vi "Firmware Wizard.vi"() -> ()   [LabVIEW 2020, in "LMH-LINX.lvlib"]
doc: "Wizard for uploading firmware to LINX devices."
uses:
  <vilib>/MakerHub/LINX/LMH-LINX.lvlib
  <vilib>/MakerHub/LINX/Private/Type Defs/Device Family.ctl
  <vilib>/MakerHub/LINX/Private/Type Defs/Devices/Device Type.ctl
  <vilib>/MakerHub/LINX/Private/Device/Type Defs/Wifi Config.ctl
  <vilib>/MakerHub/LINX/Private/Type Defs/WIFI Security Type.ctl
  <vilib>/MakerHub/LINX/Private/Type Defs/Deploy Firmware State.ctl
  <vilib>/MakerHub/LINX/Private/Type Defs/All Firmware Data FGV States.ctl
  <vilib>/MakerHub/LINX/Private/Device/Type Defs/TCP Config.ctl
  <vilib>/MakerHub/LINX/Private/Device/Type Defs/Firmware Interface.ctl
  <vilib>/MakerHub/Toolbox/LMH-Toolbox.lvlib
  <vilib>/MakerHub/LINX/Private/Device/Device.lvlib
panel:
  out "Error Out":errorcluster
  out "Log Path":path
  in  "Device Family Enum":T1 items=["National Instruments", "Digilent", "Arduino"]
  in  "Error In":errorcluster
  out "Tab Control":T2(tab)=enum."Device"
  in  "Firmware Available?":string
  in  "Settings Button":bool
  out "Device Image":picture
  in  "Device Help":bool
  in  "Device Type":T3=4 items=["Arduino Leonardo", "Arduino Mega2560", "Arduino Nano", "Arduino Pro Micro", "Arduino Uno"]
  in  "Device Family":T1 items=["Arduino", "Digilent", "PJRC", "Sparkfun"]
  in  "Device Cancel":bool
  in  "Device Next":bool
  in  "Firmware Upload Method":u16(ring) items=["Serial / USB"]
  in  "Config Message":string
  in  "Int Help":bool
  in  "Int Previous":bool
  in  "Int Cancel":bool
  in  "Int Next":bool
  out "Interface Config":enum32{"N/A", "Serial / USB", "USB", "TCP"}(tab)=enum."Serial / USB"
  in  "Upload COM Port":refnum<visa-resource-name>="ASRL1::INSTR"
  out "Firmware Configuration":enum32{"Serial", "Ethernet", "WIFI"}(tab)=enum."WIFI"
  in  "Port":u16=927
  in  "IP Address":string="192.168.1.27"
  in  "Wifi Configuration":T4
  in  "FWV Help":bool
  in  "FWV Cancel":bool
  in  "FWV Next":bool
  in  "FWV Previous":bool
  in  "Firmware Version":u16(ring) items=["LINX - Serial / USB"]
  in  "Upload Type":u16(ring) items=["Pre-Built Firmware", "Build with Arduino IDE"]
  in  "Firmware Description":string
  out "Deploy Progress Note":string
  in  "Deploy  Progress Bar":u8(slide) scale=0.0..100.0
  in  "View Log":bool
  in  "LINX Forum Link":string="www.labviewmakerhub.com/forums/linx"
  in  "LINX Landing Page Link":string="www.labviewmakerhub.com/linx"
  in  "Summary Launch Example":bool
  in  "Summary Text":string
  in  "Summary Next":bool
  in  "Summary Help":bool
  # "Ethernet Settings"
  # "WIFI Settings"
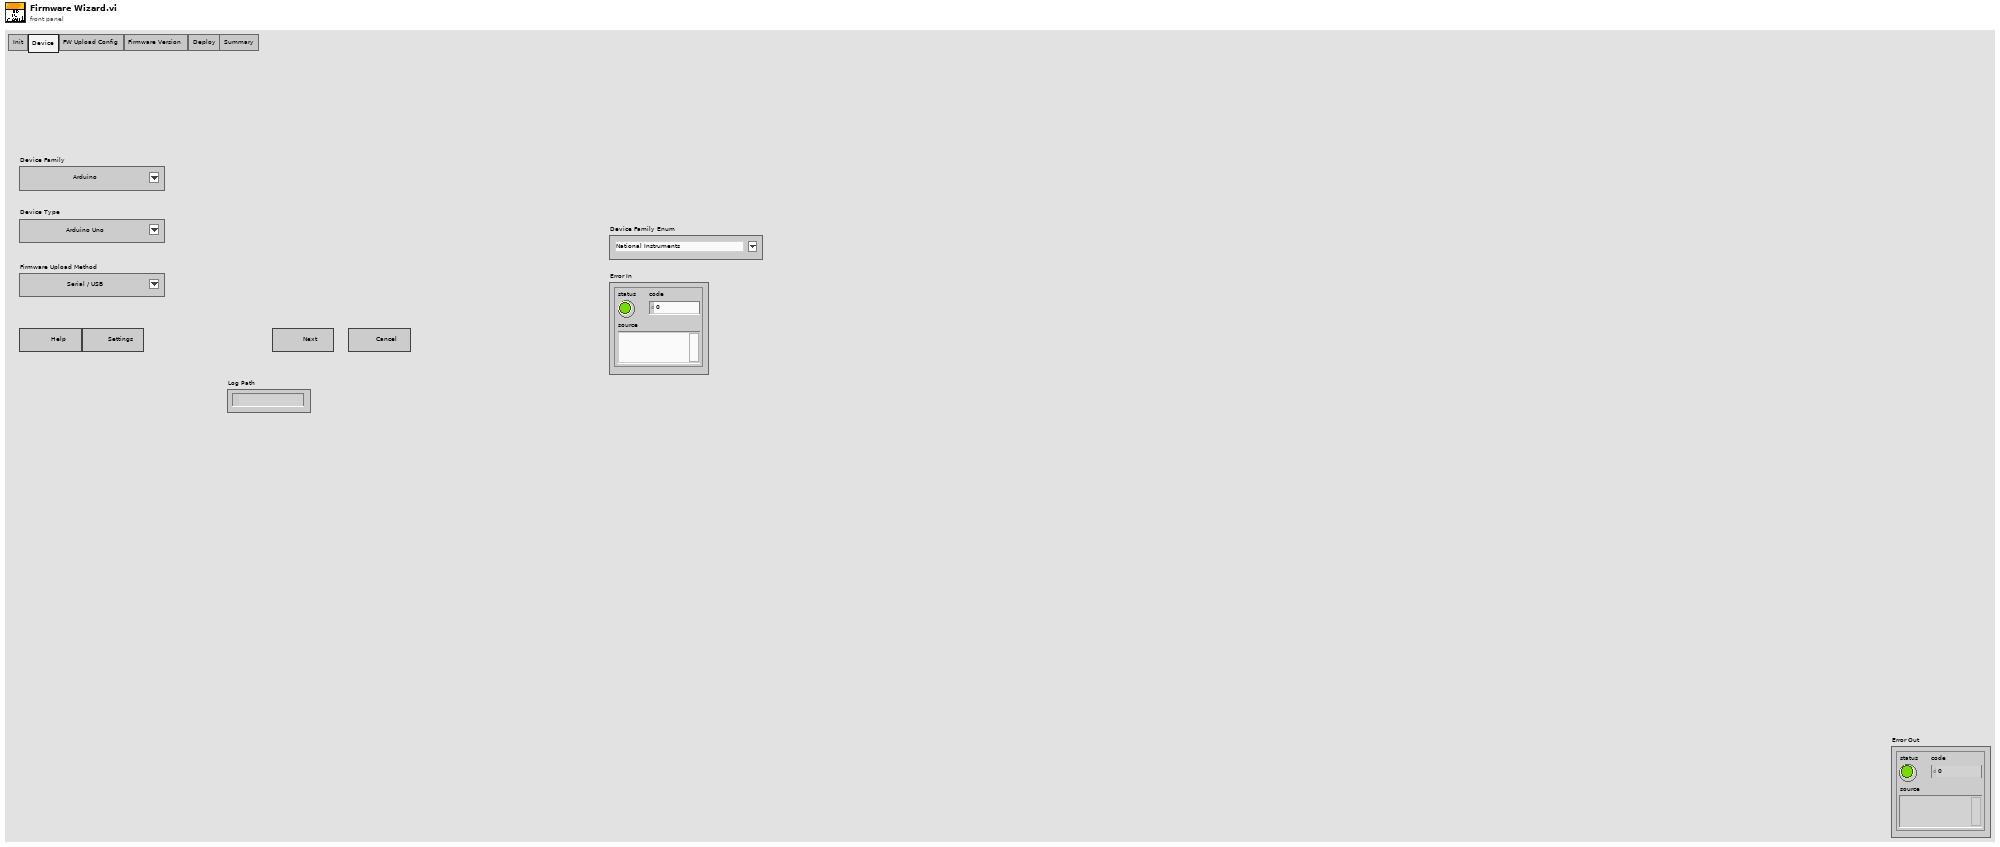
[diagram p1: front panel]
types:
  T1 = typedef "LMH-LINX.lvlib/Device Family.ctl" = u8
  T2 = enum32{"Init", "Device", "FW Upload Config", "Firmware Version", "Deploy", "Summary"}
  T3 = typedef "LMH-LINX.lvlib/Device Type.ctl" = u16
  T4 = typedef "LMH-LINX.lvlib/Device.lvlib/Wifi Config.ctl" = cluster{"SSID":string, "IP Address":string, "Port":u16, "WIFI Security Type":T5, "Password":string}
  T5 = typedef "LMH-LINX.lvlib/WIFI Security Type.ctl" = enum8{"None", "WPA2 Password", "WPA2 Key", "WEP40", "WEP104"}
  T6 = typedef "LMH-LINX.lvlib/Deploy Firmware State.ctl" = enum32{"Init", "Device", "FW Upload Config", "Firmware Version", "Deploy", "Summary"}
  T7 = typedef "LMH-LINX.lvlib/All Firmware Data FGV States.ctl" = enum16{"Set", "Get"}
  T8 = enum8{"Enabled", "Disabled", "Disabled and Grayed Out"}
  T9 = typedef "LMH-LINX.lvlib/Firmware Interface.ctl" = enum32{"Serial ", "Ethernet", "WIFI"}
  T10 = typedef "LMH-LINX.lvlib/Device.lvlib/TCP Config.ctl" = cluster{"IP Address":string, "Port":u16}
  T11 = typedef "LMH-LINX.lvlib/Device Firmware.ctl" = cluster{"Firmware Name":string, "Firmware Path":path, "Description":string, "LINX Interface":string, "Flash Util Working Dir":path, "Flash Util Name":string, "Flash Util Args":string, "Flash Timeout (ms)":i32, "Pre-Built Firmware":string, "Build with Arduino IDE":string}
  T12 = enum16{"Left Button", "Center Button", "Right Button", "Window Close"}
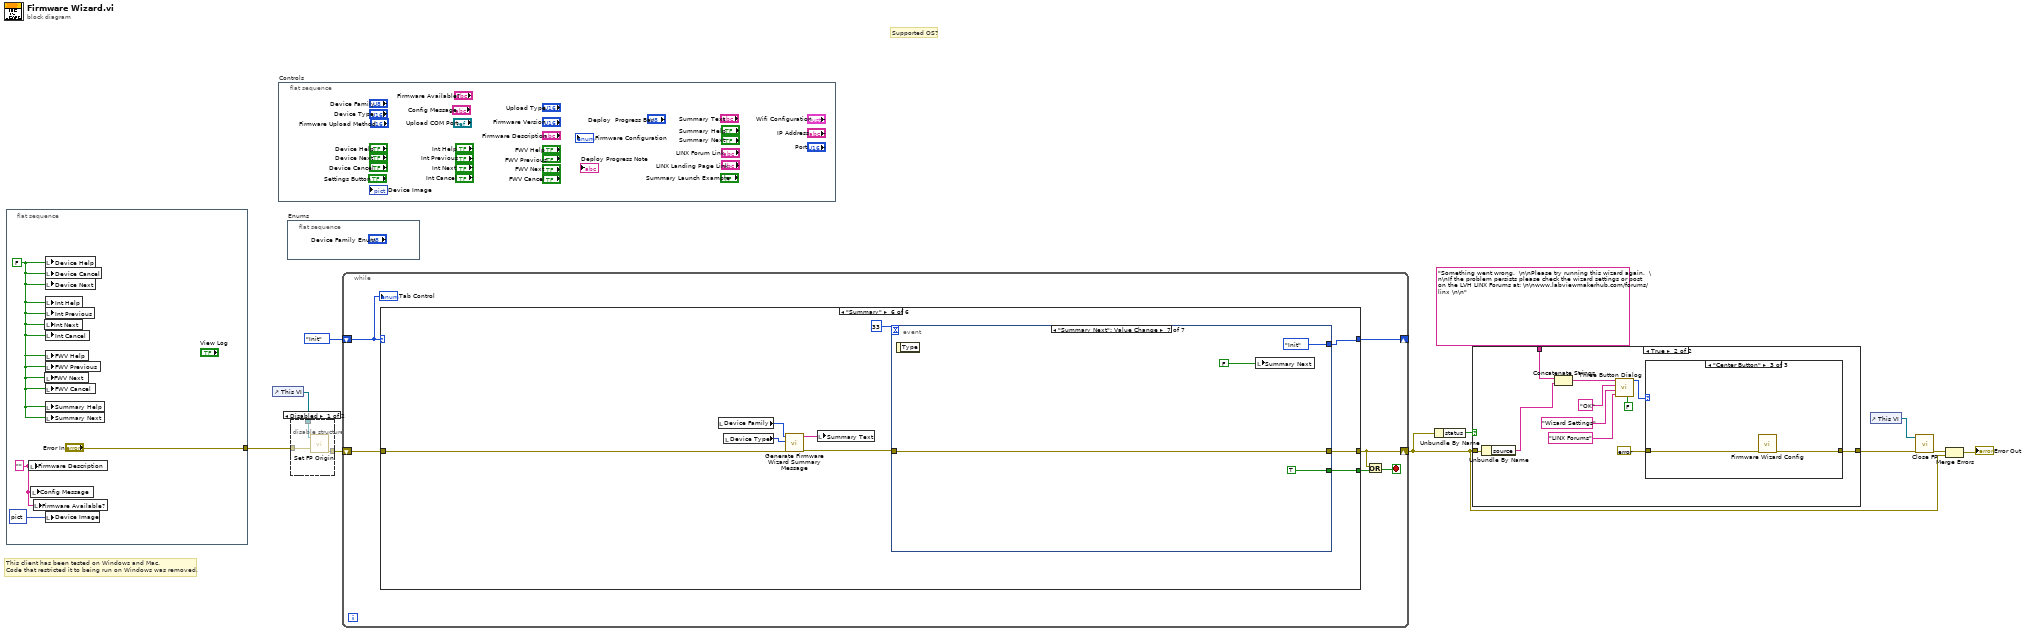
[diagram p0: block diagram]
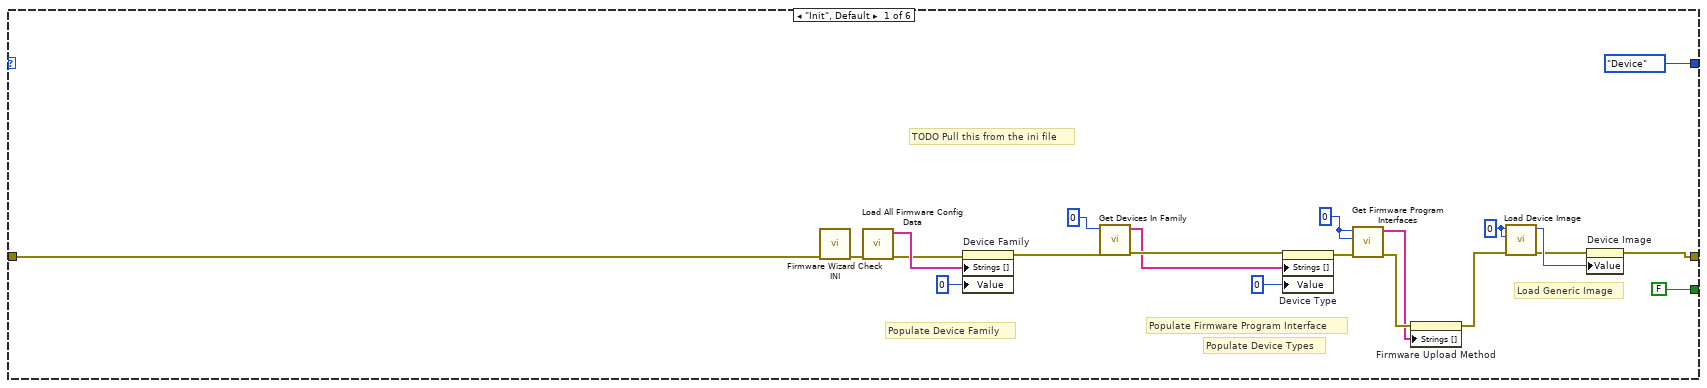
[diagram p3: hidden frame]
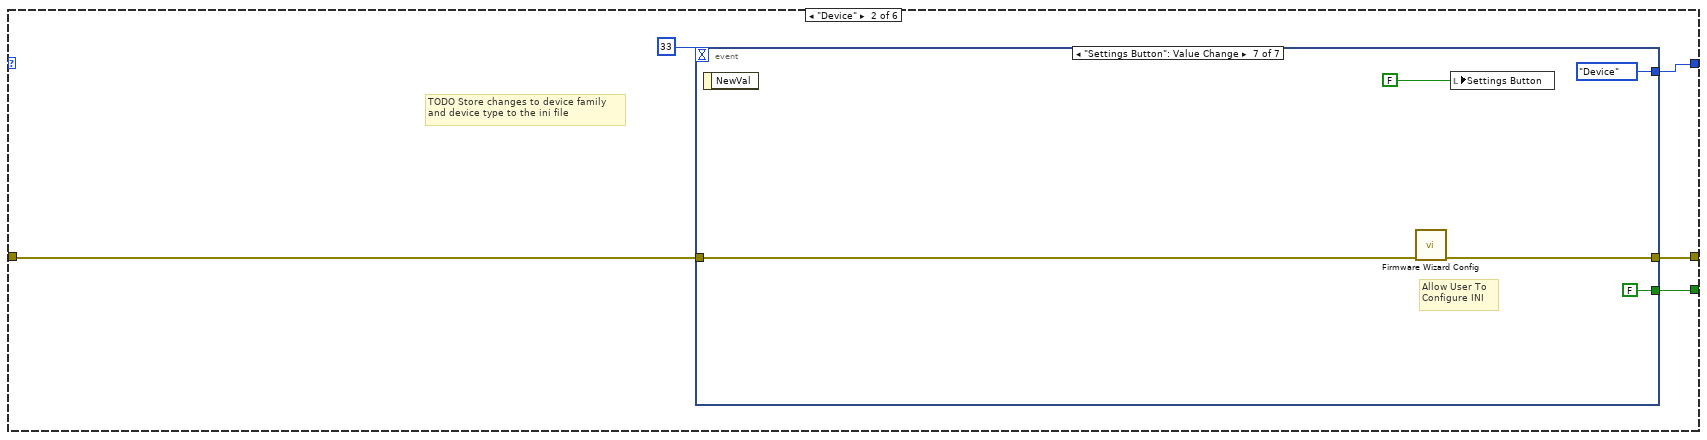
[diagram p4: hidden frame]
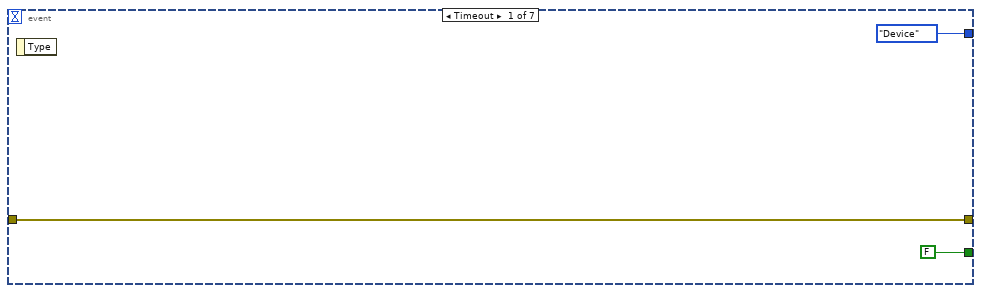
[diagram p5: hidden frame]
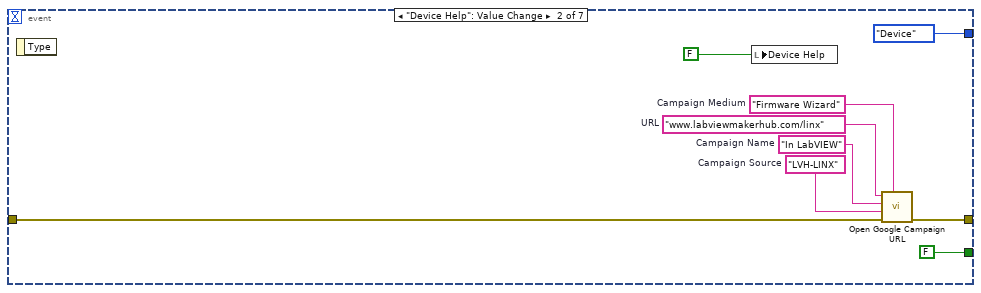
[diagram p6: hidden frame]
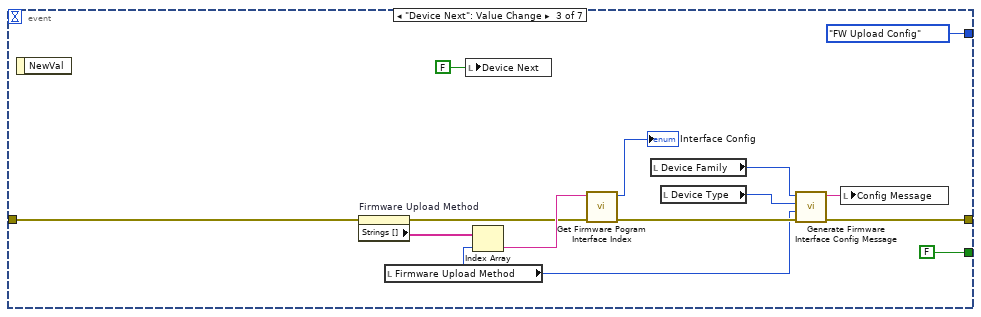
[diagram p7: hidden frame]
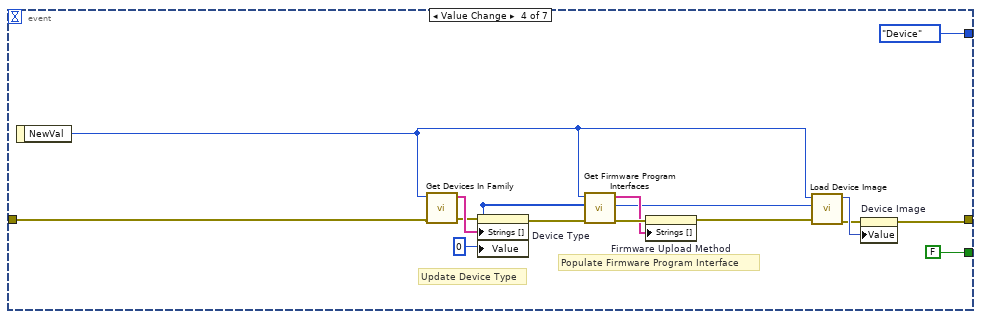
[diagram p8: hidden frame]
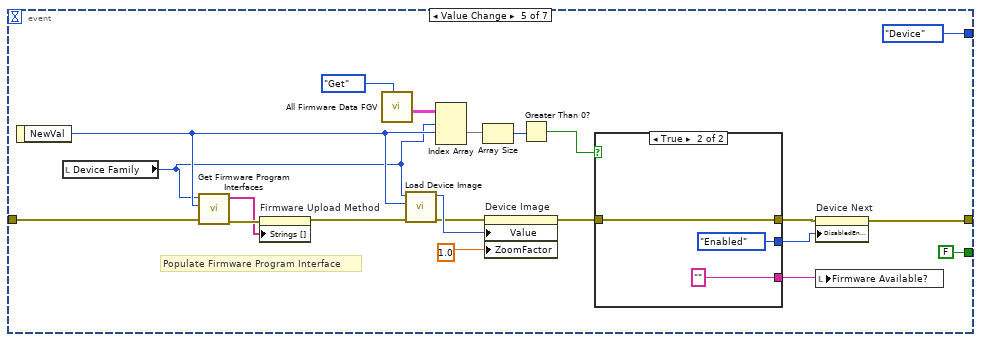
[diagram p9: hidden frame]
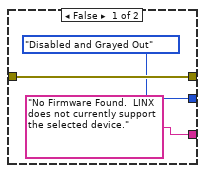
[diagram p10: hidden frame]
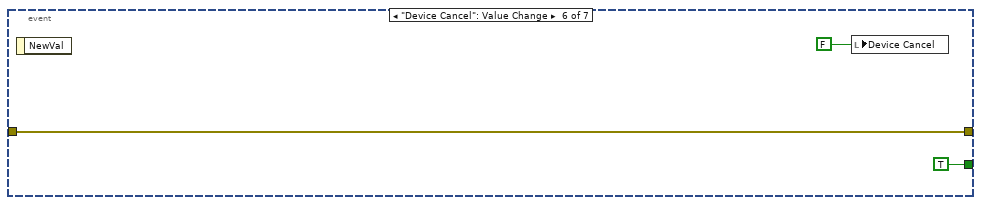
[diagram p11: hidden frame]
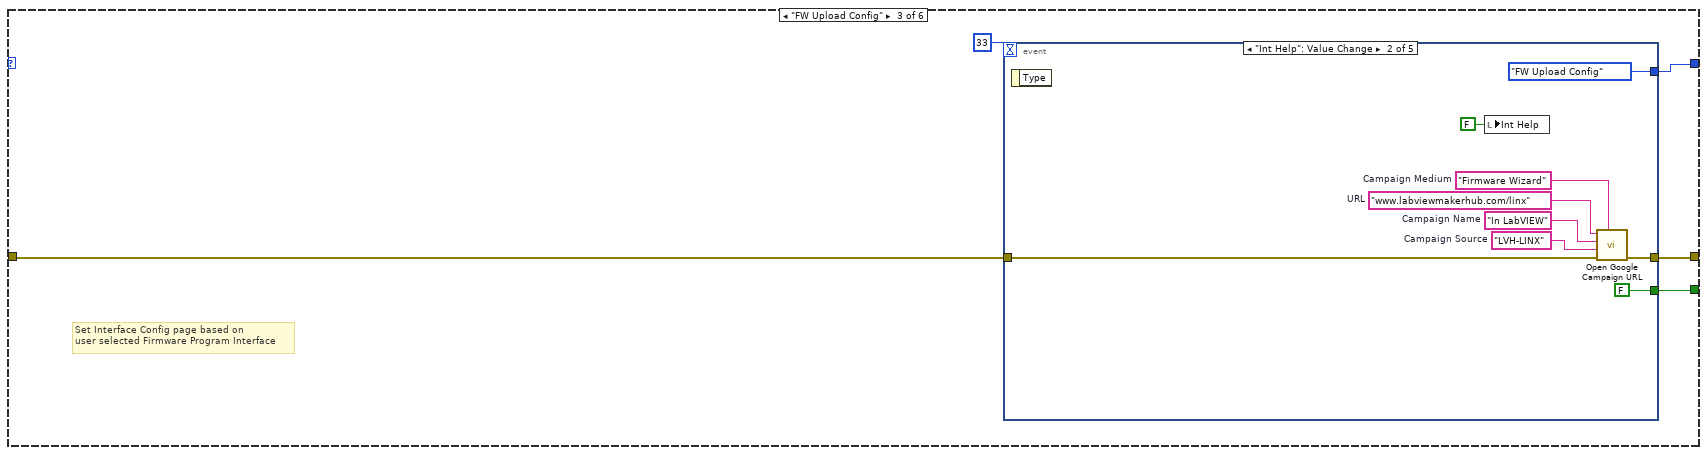
[diagram p12: hidden frame]
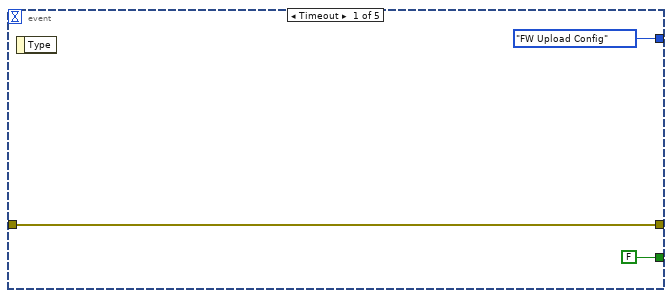
[diagram p13: hidden frame]
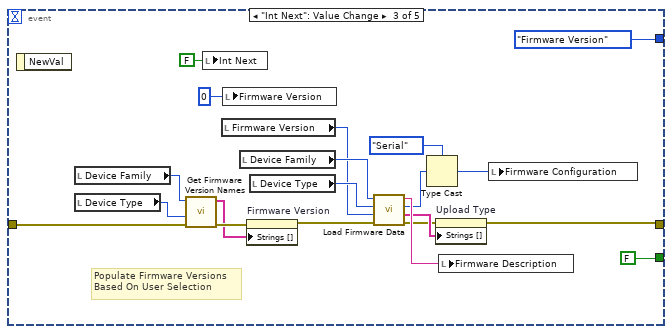
[diagram p14: hidden frame]
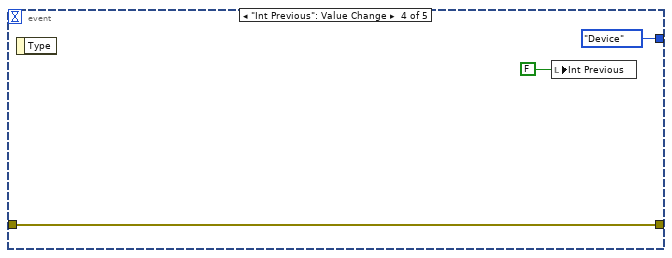
[diagram p15: hidden frame]
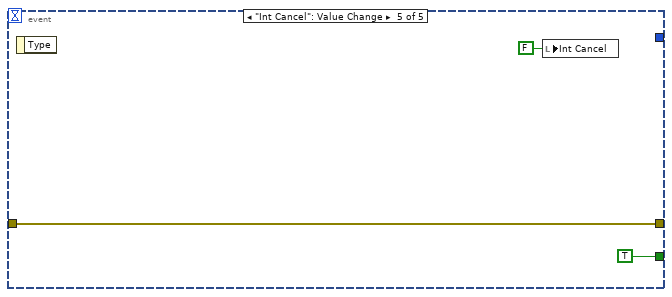
[diagram p16: hidden frame]
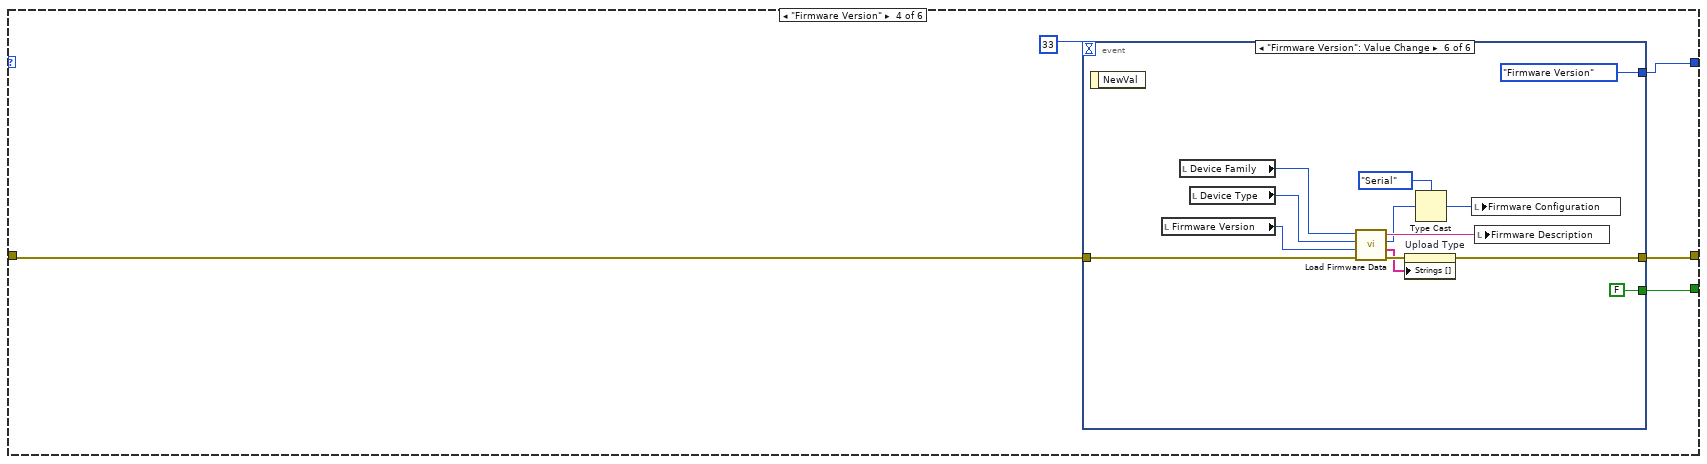
[diagram p17: hidden frame]
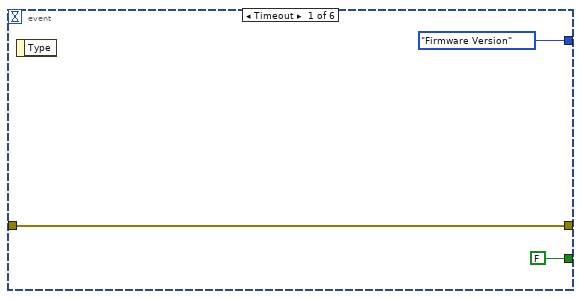
[diagram p18: hidden frame]
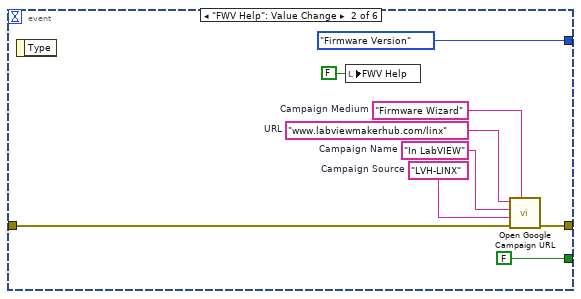
[diagram p19: hidden frame]
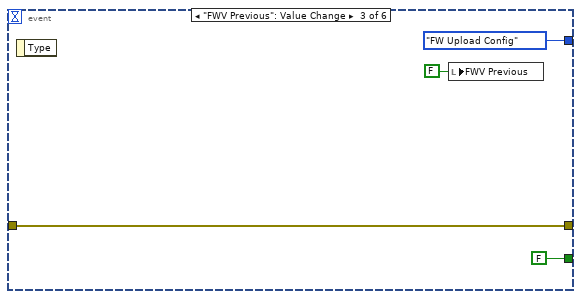
[diagram p20: hidden frame]
diagram:
  # "This client has been tested on Windows and Mac.\nCode that restricted it to being run on Windows was removed."
  # "Supported OS?"
  n1 = flat-sequence {
    tunnel: ["Error In"] -> w9
    frame #0 {
      w13 = "" ("Firmware Description")
      w15 = FALSE ("Cancel")
      n2 = local write "Firmware Description"(w13) -> ()
      n3 = local write "Config Message"(w13) -> ()
      n4 = local write "Firmware Available?"(w13) -> ()
      n5 = local write "Int Next"(w15) -> ()
      n6 = local write "FWV Next"(w15) -> ()
      n7 = local write "Device Help"(w15) -> ()
      n8 = local write "Device Cancel"(w15) -> ()
      n9 = local write "Device Next"(w15) -> ()
      n10 = local write "Int Help"(w15) -> ()
      n11 = local write "Int Previous"(w15) -> ()
      n12 = local write "Int Cancel"(w15) -> ()
      n13 = local write "FWV Help"(w15) -> ()
      n14 = local write "FWV Previous"(w15) -> ()
      n15 = local write "FWV Cancel"(w15) -> ()
      n16 = local write "Summary Help"(w15) -> ()
      n17 = local write "Summary Next"(w15) -> ()
      n18 = local write "Device Image"(picture data[5B] ("2D Picture")) -> ()
    }
  }
  n19 = control-ref of="This VI"() -> (w10:refnum<vi>)
  n20 = flat-sequence "Controls" {
    frame #0 {
    }
  }
  n21 = flat-sequence "Enums" {
    frame #0 {
    }
  }
  n22 = disable-structure shown="Disabled" {
    disable-tunnel: w10 -> [w18 _]
    disable-tunnel: w9 -> [w17 w19]
    disable-tunnel: [w16 w19] -> w8
    frame Disabled {
      n23 = call <vilib>:"Set FP Origin.vi"("Error In"=w17, "VI Ref"=w18) -> ("Error Out"=w16:errorcluster)  [unwired: 9 in]
    }
    frame Enabled {
    }
  }
  n24 = while {
    shift-right: [w23] -> _
    shift-left: Deploy_Firmware_State."Init" ("Deploy Firmware State") -> [w25]
    shift-right: [w22] -> w4
    shift-left: w8 -> [w24]
    stop <- w21 stop-if-true
    n25 = case shown="\"Summary\"" w25 {
      tunnel: [w26 w50 w130 w174 w216 w321] -> w22
      tunnel: w24 -> [w29 w49 w127 w173 w220 w317]
      tunnel: [Deploy_Firmware_State."Device" ("Deploy Firmware State") w48 w131 w171 Deploy_Firmware_State."Summary" ("Deploy Firmware State") w319] -> w23
      tunnel: [FALSE w47 w128 w170 FALSE w318] -> w20
      frame "Init", Default {
        w30 = 0 ("Device Family Index")
        w40 = 0 ("Device Family")
        # "TODO Pull this from the ini file"
        # "Load Generic Image"
        # "Populate Firmware Program Interface"
        # "Populate Device Types"
        # "Populate Device Family"
        n26 = call <vilib>:"Firmware Wizard Check INI.vi"("Error In"=w29) -> ("Error Out"=w28:errorcluster)  [unwired: 10 in]
        n27 = call <vilib>:"Load All Firmware Config Data.vi"("Error In"=w28) -> ("Error Out"=w31:errorcluster, "Families"=w32:string[])  [unwired: 7 in, 2 out]
        n28 = property on="Device Family" class="Ring (strict)"(error in=w31, "Strings []"=w32, "Value"=u16 0 ("Device Family")) -> (error out=w36:errorcluster)  [unwired: 1 in, 1 out]
        n29 = call <vilib>:"Get Devices In Family.vi"("Error In"=w36, "Family Index"=0 ("Device Family")) -> ("Error Out"=w35:errorcluster, "Devices"=w34:string[])  [unwired: 8 in]
        n30 = property on="Device Type" class="Ring (strict)"(error in=w35, "Strings []"=w34, "Value"=u16 0 ("Device Family")) -> (error out=w41:errorcluster)  [unwired: 1 in, 1 out]
        n31 = call <vilib>:"Get Firmware Program Interfaces.vi"("Error In"=w41, "Device Index"=w40, "Family Index"=w40) -> ("Error Out"=w43:errorcluster, "Firmware Program Interfaces"=w42:string[])  [unwired: 7 in]
        n32 = property on="Firmware Upload Method" class="Ring (strict)"(error in=w43, "Strings []"=w42) -> (error out=w27:errorcluster)  [unwired: 1 in, 1 out]
        n33 = call <vilib>:"Load Device Image.vi"("Error In"=w27, "Device Index"=w30, "Device Family Index"=w30) -> ("Error Out"=w37:errorcluster, "Device Image"=w38:picture)  [unwired: 6 in, 1 out]
        n34 = property on="Device Image" class="Pict"(error in=w37, "Value"=w38) -> (error out=w26:errorcluster)  [unwired: 1 in, 1 out]
      }
      frame "Device" {
        # "TODO Store changes to device family\nand device type to the ini file"
        n35 = event shown="[6] \"Settings Button\": Value Change" {
          selector: _ -> [_ _ _ _ _ _ _]
          dyn-events: _ -> [_ _ _ _ _ _ _]
          timeout: 33 -> [_ _ _ _ _ _ _]
          tunnel: [w54 w57 w74 w83 w101 w120 w123] -> w50
          tunnel: w49 -> [w54 w56 w70 w82 w112 w120 w124]
          tunnel: [Deploy_Firmware_State."Device" ("Deploy Firmware State") Deploy_Firmware_State."Device" ("Deploy Firmware State") Deploy_Firmware_State."FW Upload Config" ("Deploy Firmware State") Deploy_Firmware_State."Device" ("Deploy Firmware State") Deploy_Firmware_State."Device" ("Deploy Firmware State") _ Deploy_Firmware_State."Device" ("Deploy Firmware State")] -> w48
          tunnel: [FALSE FALSE FALSE FALSE FALSE TRUE FALSE] -> w47
          event Timeout {
            n36 = event-data() -> ()  [unwired: 1 in, 1 out]
          }
          event "Device Help": Value Change {
            w55 = "LVH-LINX"  # Campaign Source
            w58 = "In LabVIEW"  # Campaign Name
            w59 = "Firmware Wizard"  # Campaign Medium
            w60 = "www.labviewmakerhub.com/linx"  # URL
            n37 = event-data() -> ()  [unwired: 1 in, 1 out]
            n38 = local write "Device Help"(FALSE ("Device Help")) -> ()
            n39 = call <vilib>:"Open Google Campaign URL.vi"("Campaign Medium"=w59, "Error In"=w56, "Campaign Source"=w55, "Campaign Name"=w58, "URL"=w60) -> ("Error Out"=w57:errorcluster)  [unwired: 5 in, 1 out]
          }
          event "Device Next": Value Change {
            n40 = event-data() -> ()  [unwired: 1 in, 1 out]
            n41 = property on="Firmware Upload Method" class="Ring (strict)"(error in=w70) -> (error out=w71:errorcluster, "Strings []"=w73:string[])  [unwired: 1 in, 1 out]
            n42 = local read "Firmware Upload Method"() -> (w65:u16)
            n43 = local write "Device Next"(FALSE ("Next")) -> ()
            n44 = Index Array(array=w73, index=w65) -> (element=w72:string)
            n45 = call <vilib>:"Get Firmware Pogram Interface Index.vi"("Error In"=w71, "Firmware Program Interface"=w72) -> ("Error Out"=w69:errorcluster, "Interface Index"=→"Interface Config":i32)  [unwired: 8 in]
            n46 = local read "Device Family"() -> (w67:T1)
            n47 = local read "Device Type"() -> (w66:T3)
            n48 = call <vilib>:"Generate Firmware Interface Config Message.vi"("Error In"=w69, "Firmware Program Interface Index"=w65, "Device Index"=w66, "Family Index"=w67) -> ("Error Out"=w74:errorcluster, "Config Message"=w75:string)  [unwired: 6 in]
            n49 = local write "Config Message"(w75) -> ()
          }
          event Value Change {
            w78 = u16 0 ("Device Family")
            # "Populate Firmware Program Interface"
            # "Update Device Type"
            n50 = event-data() -> ("NewVal"=w79:T1)  [unwired: 1 in]
            n51 = call <vilib>:"Get Devices In Family.vi"("Error In"=w82, "Family Index"=w79) -> ("Error Out"=w80:errorcluster, "Devices"=w81:string[])  [unwired: 8 in]
            n52 = property on="Device Type" class="Ring (strict)"(error in=w80, "Strings []"=w81, "Value"=w78) -> (error out=w88:errorcluster)  [unwired: 1 in, 1 out]
            n53 = call <vilib>:"Get Firmware Program Interfaces.vi"("Error In"=w88, "Device Index"=w78, "Family Index"=w79) -> ("Error Out"=w90:errorcluster, "Firmware Program Interfaces"=w89:string[])  [unwired: 7 in]
            n54 = property on="Firmware Upload Method" class="Ring (strict)"(error in=w90, "Strings []"=w89) -> (error out=w84:errorcluster)  [unwired: 1 in, 1 out]
            n55 = call <vilib>:"Load Device Image.vi"("Error In"=w84, "Device Index"=w78, "Device Family Index"=w79) -> ("Error Out"=w85:errorcluster, "Device Image"=w86:picture)  [unwired: 6 in, 1 out]
            n56 = property on="Device Image" class="Pict"(error in=w85, "Value"=w86) -> (error out=w83:errorcluster)  [unwired: 1 in, 1 out]
          }
          event Value Change {
            # "Populate Firmware Program Interface"
            n57 = event-data() -> ("NewVal"=w93:T3)  [unwired: 1 in]
            n58 = local read "Device Family"() -> (w92:T1)
            n59 = call <vilib>:"Get Firmware Program Interfaces.vi"("Error In"=w112, "Device Index"=w93, "Family Index"=w92) -> ("Error Out"=w111:errorcluster, "Firmware Program Interfaces"=w110:string[])  [unwired: 7 in]
            n60 = property on="Firmware Upload Method" class="Ring (strict)"(error in=w111, "Strings []"=w110) -> (error out=w107:errorcluster)  [unwired: 1 in, 1 out]
            n61 = call <vilib>:"All Firmware Data FGV.vi"("All Firmware Data FGV States"=All_Firmware_Data_FGV_States."Get") -> ("Firmwares"=w98:T11[][][])  [unwired: 7 in, 3 out]
            n62 = call <vilib>:"Load Device Image.vi"("Error In"=w107, "Device Index"=w93, "Device Family Index"=w92) -> ("Error Out"=w104:errorcluster, "Device Image"=w106:picture)  [unwired: 6 in, 1 out]
            n63 = Index Array(array=w98, index (dim 0)=w92, index (dim 1)=w93) -> (element=w97:T11[])  [unwired: 1 in]
            n64 = Array Size(array=w97) -> (size(s)=w96:i32)
            n65 = property on="Device Image" class="Pict"(error in=w104, "Value"=w106, "ZoomFactor"=sgl 1.0 ("Zoom Factor")) -> (error out=w103:errorcluster)  [unwired: 1 in, 1 out]
            n66 = Greater Than 0?(x=w96) -> (x > 0?=w95:bool)
            n67 = case shown="True" w95 {
              tunnel: [w115 w118] -> w102
              tunnel: w103 -> [w115 w118]
              tunnel: [T8."Disabled and Grayed Out" ("Disabled") T8."Enabled" ("Disabled")] -> w100
              tunnel: ["No Firmware Found.  LINX does not currently support the selected device." ("Firmware Available?") "" ("Firmware Available?")] -> w99
              frame False {
              }
              frame True {
              }
            }
            n68 = property on="Device Next" class="Bool (strict)"(error in=w102, "DisabledEnum"=w100) -> (error out=w101:errorcluster)  [unwired: 1 in, 1 out]
            n69 = local write "Firmware Available?"(w99) -> ()
          }
          event "Device Cancel": Value Change {
            n70 = event-data() -> ()  [unwired: 1 in, 1 out]
            n71 = local write "Device Cancel"(FALSE ("Device Cancel")) -> ()
          }
          event "Settings Button": Value Change {
            # "Allow User To \nConfigure INI"
            n72 = event-data() -> ()  [unwired: 1 in, 1 out]
            n73 = call <vilib>:"Firmware Wizard Config.vi"("Error In"=w124) -> ("Error Out"=w123:errorcluster)  [unwired: 10 in]
            n74 = local write "Settings Button"(FALSE ("Settings Button")) -> ()
          }
        }
      }
      frame "FW Upload Config" {
        # "Set Interface Config page based on \nuser selected Firmware Program Interface"
        n75 = event shown="[1] \"Int Help\": Value Change" {
          selector: _ -> [_ _ _ _ _]
          dyn-events: _ -> [_ _ _ _ _]
          timeout: 33 -> [_ _ _ _ _]
          tunnel: [Deploy_Firmware_State."FW Upload Config" ("Deploy Firmware State") Deploy_Firmware_State."FW Upload Config" ("Deploy Firmware State") Deploy_Firmware_State."Firmware Version" ("Deploy Firmware State") Deploy_Firmware_State."Device" ("Deploy Firmware State") _] -> w131
          tunnel: [w133 w135 w144 w166 w167] -> w130
          tunnel: w127 -> [w133 w136 w163 w166 w167]
          tunnel: [FALSE FALSE FALSE _ TRUE] -> w128
          event Timeout {
            n76 = event-data() -> ()  [unwired: 1 in, 1 out]
          }
          event "Int Help": Value Change {
            w137 = "LVH-LINX"  # Campaign Source
            w138 = "In LabVIEW"  # Campaign Name
            w139 = "Firmware Wizard"  # Campaign Medium
            w140 = "www.labviewmakerhub.com/linx"  # URL
            n77 = event-data() -> ()  [unwired: 1 in, 1 out]
            n78 = local write "Int Help"(FALSE ("Int Help")) -> ()
            n79 = call <vilib>:"Open Google Campaign URL.vi"("Campaign Medium"=w139, "Error In"=w136, "Campaign Source"=w137, "Campaign Name"=w138, "URL"=w140) -> ("Error Out"=w135:errorcluster)  [unwired: 5 in, 1 out]
          }
          event "Int Next": Value Change {
            # "Populate Firmware Versions\nBased On User Selection"
            n80 = event-data() -> ()  [unwired: 1 in, 1 out]
            n81 = local read "Device Family"() -> (w159:T1)
            n82 = local read "Device Type"() -> (w160:T3)
            n83 = call <vilib>:"Get Firmware Version Names.vi"("Error In"=w163, "Device Index"=w160, "Family Index"=w159) -> ("Error Out"=w162:errorcluster, "Firmware Version Names"=w161:string[])  [unwired: 6 in, 1 out]
            n84 = local write "Int Next"(FALSE ("Int Next")) -> ()
            n85 = local read "Firmware Version"() -> (w148:u16)
            n86 = local write "Firmware Version"(0) -> ()
            n87 = local read "Device Family"() -> (w150:T1)
            n88 = property on="Firmware Version" class="Ring (strict)"(error in=w162, "Strings []"=w161) -> (error out=w154:errorcluster)  [unwired: 1 in, 1 out]
            n89 = local read "Device Type"() -> (w149:T3)
            n90 = call <vilib>:"Load Firmware Data.vi"("Error In"=w154, "Firmware Index"=w148, "Device Index"=w149, "Family Index"=w150) -> ("Error Out"=w145:errorcluster, "Upload Type"=w146:string[], "Firmware Interface"=w147:T9, "Firmware Description"=w155:string)  [unwired: 4 in]
            n91 = Type Cast(type=enum32{"Serial", "Ethernet", "WIFI"}."Serial" ("Firmware Configuration"), x=w147) -> (*(type *) &x=w151:enum32{"Serial", "Ethernet", "WIFI"})
            n92 = property on="Upload Type" class="Ring (strict)"(error in=w145, "Strings []"=w146) -> (error out=w144:errorcluster)  [unwired: 1 in, 1 out]
            n93 = local write "Firmware Description"(w155) -> ()
            n94 = local write "Firmware Configuration"(w151) -> ()
          }
          event "Int Previous": Value Change {
            n95 = event-data() -> ()  [unwired: 1 in, 1 out]
            n96 = local write "Int Previous"(FALSE ("Previous")) -> ()
          }
          event "Int Cancel": Value Change {
            n97 = event-data() -> ()  [unwired: 1 in, 1 out]
            n98 = local write "Int Cancel"(FALSE ("Int Cancel")) -> ()
          }
        }
      }
      frame "Firmware Version" {
        n99 = event shown="[5] \"Firmware Version\": Value Change" {
          selector: _ -> [_ _ _ _ _ _]
          dyn-events: _ -> [_ _ _ _ _ _]
          timeout: 33 -> [_ _ _ _ _ _]
          tunnel: [w177 w179 w189 w193 w197 w200] -> w174
          tunnel: w173 -> [w177 w178 w189 w193 w197 w209]
          tunnel: [Deploy_Firmware_State."Firmware Version" ("Deploy Firmware State") Deploy_Firmware_State."Firmware Version" ("Deploy Firmware State") Deploy_Firmware_State."FW Upload Config" ("Deploy Firmware State") Deploy_Firmware_State."Deploy" ("Deploy Firmware State") Deploy_Firmware_State."Init" ("Deploy Firmware State") Deploy_Firmware_State."Firmware Version" ("Deploy Firmware State")] -> w171
          tunnel: [FALSE FALSE FALSE FALSE TRUE FALSE] -> w170
          event Timeout {
            n100 = event-data() -> ()  [unwired: 1 in, 1 out]
          }
          event "FWV Help": Value Change {
            w180 = "LVH-LINX"  # Campaign Source
            w181 = "In LabVIEW"  # Campaign Name
            w182 = "Firmware Wizard"  # Campaign Medium
            w183 = "www.labviewmakerhub.com/linx"  # URL
            n101 = event-data() -> ()  [unwired: 1 in, 1 out]
            n102 = local write "FWV Help"(FALSE ("FWV Help")) -> ()
            n103 = call <vilib>:"Open Google Campaign URL.vi"("Campaign Medium"=w182, "Error In"=w178, "Campaign Source"=w180, "Campaign Name"=w181, "URL"=w183) -> ("Error Out"=w179:errorcluster)  [unwired: 5 in, 1 out]
          }
          event "FWV Previous": Value Change {
            n104 = event-data() -> ()  [unwired: 1 in, 1 out]
            n105 = local write "FWV Previous"(FALSE ("FWV Previous")) -> ()
          }
          event "FWV Next": Value Change {
            n106 = event-data() -> ()  [unwired: 1 in, 1 out]
            n107 = local write "FWV Next"(FALSE ("FWV Previous")) -> ()
          }
          event "FWV Cancel": Value Change {
            n108 = event-data() -> ()  [unwired: 1 in, 1 out]
            n109 = local write "FWV Cancel"(FALSE ("FWV Previous")) -> ()
          }
          event "Firmware Version": Value Change {
            n110 = event-data() -> ()  [unwired: 1 in, 1 out]
            n111 = local read "Firmware Version"() -> (w202:u16)
            n112 = local read "Device Family"() -> (w204:T1)
            n113 = local read "Device Type"() -> (w203:T3)
            n114 = call <vilib>:"Load Firmware Data.vi"("Error In"=w209, "Firmware Index"=w202, "Device Index"=w203, "Family Index"=w204) -> ("Error Out"=w201:errorcluster, "Upload Type"=w199:string[], "Firmware Interface"=w206:T9, "Firmware Description"=w208:string)  [unwired: 4 in]
            n115 = property on="Upload Type" class="Ring (strict)"(error in=w201, "Strings []"=w199) -> (error out=w200:errorcluster)  [unwired: 1 in, 1 out]
            n116 = Type Cast(type=enum32{"Serial", "Ethernet", "WIFI"}."Serial" ("Firmware Configuration"), x=w206) -> (*(type *) &x=w205:enum32{"Serial", "Ethernet", "WIFI"})
            n117 = local write "Firmware Configuration"(w205) -> ()
            n118 = local write "Firmware Description"(w208) -> ()
          }
        }
      }
      frame "Deploy" {
        n119 = flat-sequence {
          tunnel: w220 -> [w230]
          tunnel: [w229] -> w219
          tunnel: [w231] -> w215
          tunnel: [w228] -> w214
          tunnel: [w226] -> w213
          tunnel: [w277] -> w222
          tunnel: [w276] -> w221
          tunnel: w219 -> [w275]
          tunnel: w215 -> [w272]
          tunnel: w214 -> [w273]
          tunnel: w213 -> [w270]
          tunnel: "Verifying and Uploading with Arduino IDE (This May Take Over 30 Seconds Depending on Your Computer)" ("Deploy Progress Note") -> [w267]
          tunnel: w222 -> [w300]
          tunnel: w221 -> [w299]
          tunnel: [w300] -> w218
          tunnel: [w299] -> w217
          tunnel: w218 -> [w309]
          tunnel: w217 -> [w308]
          tunnel: [w303] -> w216
          frame #0 {
            n120 = local read "Upload Type"() -> (w227:u16)
            n121 = local write "Deploy Progress Note"("Verifying Upload Type" ("Deploy Progress Note")) -> ()
            n122 = case shown="1" w227 {
              selector: w227 -> [_ w240]
              tunnel: [w234 w248] -> w231
              tunnel: w227 -> [_ w247]
              tunnel: w230 -> [w235 w246]
              tunnel: [w235 w242] -> w229
              tunnel: [w234 w244] -> w228
              tunnel: [FALSE w237] -> w226
              tunnel: "Arduino IDE Path Is Missing Or LINX Libraries Were Not Found" -> [_ w236]
              frame 0, Default {
                w234 = path ""
              }
              frame 1 {
                n123 = call <vilib>:"Check For Empty Path.vi"("Error In"=w246, "Upload Type"=w247) -> ("Error Out"=w245:errorcluster, "Good Paths?"=w239:bool, "Arduino Base Path"=w244:path, "Firmware Builds Base Path"=w248:path)  [unwired: 6 in]
                n124 = call <vilib>:"Verify Arduino Libraries.vi"("Error In"=w245, "Arduino Base Path"=w244) -> ("Error Out"=w243:errorcluster, "Libraries Exst?"=w238:bool)  [unwired: 7 in, 1 out]
                n125 = And(x=w238, y=w239) -> (x .and. y?=w241:bool)
                n126 = case shown="False" w241 {
                  tunnel: w243 -> [w259 w266]
                  tunnel: [w251 w266] -> w242
                  tunnel: w241 -> [_ w265]
                  tunnel: w240 -> [w257 _]
                  tunnel: [w250 w265] -> w237
                  tunnel: w236 -> [w249 _]
                  frame False {
                    n127 = call <vilib>:"Firmware Wizard Config.vi"("Error In"=w259) -> ("Error Out"=w258:errorcluster)  [unwired: 10 in]
                    n128 = call <vilib>:"Check For Empty Path.vi"("Error In"=w258, "Upload Type"=w257) -> ("Error Out"=w255:errorcluster, "Good Paths?"=w253:bool, "Arduino Base Path"=w256:path)  [unwired: 6 in, 1 out]
                    n129 = call <vilib>:"Verify Arduino Libraries.vi"("Error In"=w255, "Arduino Base Path"=w256) -> ("Error Out"=w252:errorcluster, "Libraries Exst?"=w254:bool)  [unwired: 7 in, 1 out]
                    n130 = And(x=w254, y=w253) -> (x .and. y?=w250:bool)
                    n131 = case shown="False" w250 {
                      tunnel: w252 -> [w263 w264]
                      tunnel: [w262 w264] -> w251
                      tunnel: w249 -> [w260 _]
                      frame False {
                        n132 = call <vilib>:"Error Cluster From Error Code.vi"("error in (no error)"=w263, "error message (\"\")"=w260, "error code (0)"=5999) -> ("error out"=w262:errorcluster)  [unwired: 6 in]
                        n133 = One Button Dialog(message=w260) -> ()  [unwired: 1 in, 1 out]
                      }
                      frame True {
                      }
                    }
                  }
                  frame True {
                  }
                }
              }
            }
          }
          frame #1 {
            n134 = local read "Upload COM Port"() -> (w276:refnum<visa-resource-name>)
            n135 = local read "Firmware Version"() -> (w274:u16)
            n136 = local read "Device Family"() -> (w279:T1)
            n137 = local read "Device Type"() -> (w278:T3)
            n138 = control-ref of="Deploy  Progress Bar"() -> (w280:refnum<vi>)
            n139 = Select(t=w267, s=w270, f="Uploading Pre-Built Hex" ("Deploy Progress Note")) -> (s? t:f=w268:string)
            n140 = case shown="True" w270 {
              tunnel: w280 -> [w288 w292]
              tunnel: w279 -> [w287 w294]
              tunnel: w278 -> [w286 w295]
              tunnel: [w285 w298] -> w277
              tunnel: w276 -> [w284 w293]
              tunnel: w275 -> [w283 w297]
              tunnel: w274 -> [w282 w296]
              tunnel: w273 -> [_ w291]
              tunnel: w272 -> [_ w290]
              tunnel: [w281 w289] -> w271
              frame False {
                n141 = call <vilib>:"Upload Firmware.vi"("Progress Bar"=w288, "COM Port"=w284, "Error In"=w283, "Firmware Index"=w282, "Device Index"=w286, "Family Index"=w287) -> ("Error Out"=w285:errorcluster, "Log Path"=w281:path)  [unwired: 4 in]
              }
              frame True {
                n142 = call <vilib>:"CommandLineUploadWizardInt.vi"("Arduino Base Path"=w291, "Progress Bar"=w292, "Firmware Base Path"=w290, "Upload COM Port"=w293, "Error In"=w297, "Firmware Version"=w296, "Device Type"=w295, "Device Family"=w294) -> ("Error Out"=w298:errorcluster, "Log Path"=w289:path)  [unwired: 2 in]
              }
            }
            "Log Path" <- w271
            n143 = local write "Deploy Progress Note"(w268) -> ()
          }
          frame #2 {
            n144 = local write "Deploy Progress Note"("Configuring Device Settings" ("Deploy Progress Note")) -> ()
          }
          frame #3 {
            n145 = local read "IP Address"() -> (w312:string)
            n146 = local read "Firmware Configuration"() -> (w305:enum32{"Serial", "Ethernet", "WIFI"})
            n147 = local read "Port"() -> (w311:u16)
            n148 = local read "Wifi Configuration"() -> (w302:T4)
            n149 = Bundle By Name(cluster=T10 {"IP Address"="", "Port"=0} ("TCP Configuration"), "IP Address"=w312, "Port"=w311) -> (w307:T10)
            n150 = Type Cast(type=Firmware_Interface."Serial " ("Firmware Interface"), x=w305) -> (*(type *) &x=w306:T9)
            n151 = call <vilib>:"Configure LINX Device.vi"("Wifi Configuration"=w302, "TCP Configuration"=w307, "Error In"=w309, "Firmware Interface"=w306, "COM Port"=w308) -> ("Error Out"=w303:errorcluster)  [unwired: 6 in]
          }
        }
      }
      frame "Summary" {
        n152 = local read "Device Family"() -> (w315:T1)
        n153 = local read "Device Type"() -> (w314:T3)
        n154 = call <vilib>:"Generate Firmware Wizard Summary Message.vi"("Error In"=w317, "Device ID"=w314, "Device Family"=w315) -> ("Error Out"=w316:errorcluster, "Summary"=w313:string)  [unwired: 7 in]
        n155 = local write "Summary Text"(w313) -> ()
        n156 = event shown="[6] \"Summary Next\": Value Change" {
          selector: _ -> [_ _ _ _ _ _ _]
          dyn-events: _ -> [_ _ _ _ _ _ _]
          timeout: 33 -> [_ _ _ _ _ _ _]
          tunnel: [w324 w331 w338 w346 w347 w366 w383] -> w321
          tunnel: w316 -> [w324 w330 w337 w345 w348 w359 w383]
          tunnel: [Deploy_Firmware_State."Summary" ("Deploy Firmware State") Deploy_Firmware_State."Summary" ("Deploy Firmware State") Deploy_Firmware_State."Summary" ("Deploy Firmware State") Deploy_Firmware_State."Summary" ("Deploy Firmware State") Deploy_Firmware_State."Summary" ("Deploy Firmware State") Deploy_Firmware_State."Summary" ("Deploy Firmware State") Deploy_Firmware_State."Init" ("Deploy Firmware State")] -> w319
          tunnel: [FALSE _ _ _ _ TRUE TRUE] -> w318
          event Timeout {
            n157 = event-data() -> ()  [unwired: 1 in, 1 out]
          }
          event "LINX Forum Link": Mouse Down {
            w326 = "LVH-LINX"  # Campaign Source
            w327 = "In LabVIEW"  # Campaign Name
            w328 = "Firmware Wizard"  # Campaign Medium
            w329 = "www.labviewmakerhub.com/forums/linx"  # URL
            n158 = event-data() -> ()  [unwired: 1 in, 7 out]
            n159 = call <vilib>:"Open Google Campaign URL.vi"("Campaign Medium"=w328, "Error In"=w330, "Campaign Source"=w326, "Campaign Name"=w327, "URL"=w329) -> ("Error Out"=w331:errorcluster)  [unwired: 5 in, 1 out]
          }
          event "LINX Landing Page Link": Mouse Down {
            w333 = "LVH-LINX"  # Campaign Source
            w334 = "In LabVIEW"  # Campaign Name
            w335 = "Firmware Wizard"  # Campaign Medium
            w336 = "www.labviewmakerhub.com/linx"  # URL
            n160 = event-data() -> ()  [unwired: 1 in, 7 out]
            n161 = call <vilib>:"Open Google Campaign URL.vi"("Campaign Medium"=w335, "Error In"=w337, "Campaign Source"=w333, "Campaign Name"=w334, "URL"=w336) -> ("Error Out"=w338:errorcluster)  [unwired: 5 in, 1 out]
          }
          event "Summary Help": Value Change {
            w341 = "LVH-LINX"  # Campaign Source
            w342 = "In LabVIEW"  # Campaign Name
            w343 = "Firmware Wizard"  # Campaign Medium
            w344 = "www.labviewmakerhub.com/linx"  # URL
            n162 = event-data() -> ()  [unwired: 1 in, 1 out]
            n163 = local write "Summary Help"(FALSE ("Summary Help")) -> ()
            n164 = call <vilib>:"Open Google Campaign URL.vi"("Campaign Medium"=w343, "Error In"=w345, "Campaign Source"=w341, "Campaign Name"=w342, "URL"=w344) -> ("Error Out"=w346:errorcluster)  [unwired: 5 in, 1 out]
          }
          event "View Log": Value Change {
            w355 = "\"" ("string")
            # "Open Log File In Default Text Editor"
            n165 = event-data() -> ()  [unwired: 1 in, 5 out]
            n166 = local read "Log Path"() -> (w350:path)
            n167 = Path To String(path=w350) -> (string=w356:string)
            n168 = Concatenate Strings("cmd /k" ("command line"), w355, w356, w355) -> (w353:string)
            n169 = local write "View Log"(FALSE ("Summary Help")) -> ()
            n170 = call <vilib>:"System Exec.vi"("run minimized? (F)"=TRUE, "wait until completion? (T)"=FALSE, "command line"=w353) -> ("error out"=w349:errorcluster)  [unwired: 5 in, 3 out]
            n171 = Merge Errors(w349, w348) -> (w347:errorcluster)
          }
          event "Summary Launch Example": Value Change {
            n172 = event-data() -> ()  [unwired: 1 in, 1 out]
            n173 = local read "Firmware Configuration"() -> (w376:enum32{"Serial", "Ethernet", "WIFI"})
            n174 = Type Cast(type=Firmware_Interface."Serial " ("Firmware Interface"), x=w376) -> (*(type *) &x=w374:T9)
            n175 = case shown="\"Ethernet\", \"WIFI\"" w374 {
              tunnel: ["LINX - Blink (Simple).vi" ("name or relative path") "LINX - Blink (Simple) (TCP).vi" ("name or relative path")] -> w363
              frame "Serial ", Default {
              }
              frame "Ethernet", "WIFI" {
              }
            }
            n176 = local write "Summary Launch Example"(FALSE ("Summary Launch Example")) -> ()
            n177 = call <vilib>:"Get Current LV Dir.vi"("Error In"=w359) -> ("Error Out"=w360:errorcluster, "This LV Directory"=w361:path)  [unwired: 9 in]
            n178 = call <vilib>:"Append Relative Path String.vi"("Error In"=w360, "Relative Path"="\\examples\\MakerHub\\LINX", "Base Path"=w361) -> ("Error Out"=w365:errorcluster, "Absolute Path"=w364:path)  [unwired: 7 in]
            n179 = Build Path(base path=w364, name or relative path=w363) -> (appended path=w372:path)
            n180 = Open VI Reference(vi path=w372, error in (no error)=w365) -> (vi reference=w371:refnum<vi>, error out=w370:errorcluster)  [unwired: 4 in]
            n181 = property class="VI"(reference=w371, error in=w370, "Front Panel.Open"=TRUE ("Front Panel Window:Open")) -> (reference out=w367:refnum<vi>, error out=w368:errorcluster)
            n182 = Close Reference(reference=w367, error in (no error)=w368) -> (error out=w366:errorcluster)
          }
          event "Summary Next": Value Change {
            n183 = event-data() -> ()  [unwired: 1 in, 1 out]
            n184 = local write "Summary Next"(FALSE ("FWV Previous")) -> ()
          }
        }
      }
    }
    n185 = Or(x=w22, y=w20) -> (x .or. y?=w21:bool)
    "Tab Control" <- w25
  }
  n186 = Unbundle By Name(w4) -> ("status"=w7:bool)
  n187 = case shown="True" w7 {
    tunnel: [w385 w395] -> w2
    tunnel: w4 -> [w385 w388]
    tunnel: "Something went wrong.  \n\nPlease try running this wizard again.  \n\nIf the problem persists please check the wizard settings or post on the LVH LINX Forums at: \n\nwww.labviewmakerhub.com/forums/linx \n\n" -> [_ w386]
    frame False {
    }
    frame True {
      n188 = Unbundle By Name(w388) -> ("source"=w387:string)
      n189 = Concatenate Strings(w386, w387) -> (w389:string)
      n190 = call <vilib>:"Three Button Dialog.vi"("Allow user to close window? (TRUE)"=FALSE, "Right Button Text (\"Cancel\")"="LINX Forums" ("F button name (\"Cancel\")"), "Center Button Text (\"No\")"="Wizard Settings" ("F button name (\"Cancel\")"), "Left Button Text (\"Yes\")"="OK" ("Left Button Text (\"Yes\")"), "message"=w389) -> ("Which Button?"=w390:T12)  [unwired: 6 in]
      n191 = case shown="\"Center Button\"" w390 {
        tunnel: errorcluster {"status"=FALSE, "code"=0, "source"=""} ("error constant") -> [w397 w399 w405]
        tunnel: [w397 w398 w404] -> w395
        frame "Left Button", Default {
          # "Nothing To Do Here"
        }
        frame "Right Button" {
          w400 = "LVH-LINX"  # Campaign Source
          w401 = "In LabVIEW"  # Campaign Name
          w402 = "Firmware Wizard"  # Campaign Medium
          w403 = "www.labviewmakerhub.com/forums/linx"  # URL
          # "Visit Forums"
          n192 = call <vilib>:"Open Google Campaign URL.vi"("Campaign Medium"=w402, "Error In"=w399, "Campaign Source"=w400, "Campaign Name"=w401, "URL"=w403) -> ("Error Out"=w398:errorcluster)  [unwired: 5 in, 1 out]
        }
        frame "Center Button" {
          n193 = call <vilib>:"Firmware Wizard Config.vi"("Error In"=w405) -> ("Error Out"=w404:errorcluster)  [unwired: 10 in]
        }
      }
    }
  }
  n194 = control-ref of="This VI"() -> (w6:refnum<vi>)
  n195 = call <vilib>:"Close FP.vi"("Error In"=w2, "VI Ref"=w6) -> ("Error Out"=w5:errorcluster)  [unwired: 9 in]
  n196 = Merge Errors(w5, w4) -> (→"Error Out":errorcluster)
